vi "2.1.vi"() -> ()   [LabVIEW 2020]
uses:
  <vilib>/numeric/Random Number (Range) U64.vi
  <vilib>/numeric/sub_Random U32.vi
panel:
  out "Array 2":dbl[][](array[numeric])
  in  "Array":dbl[][](array[numeric])
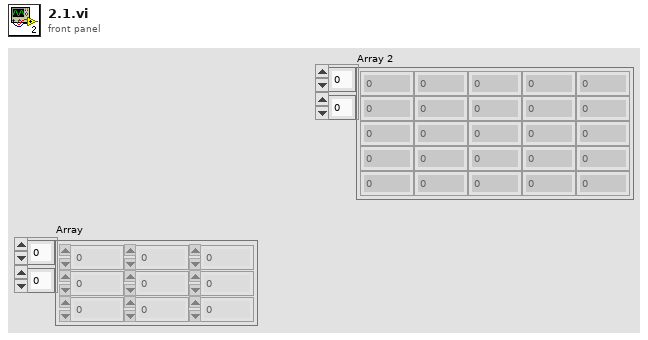
[diagram p1: front panel]
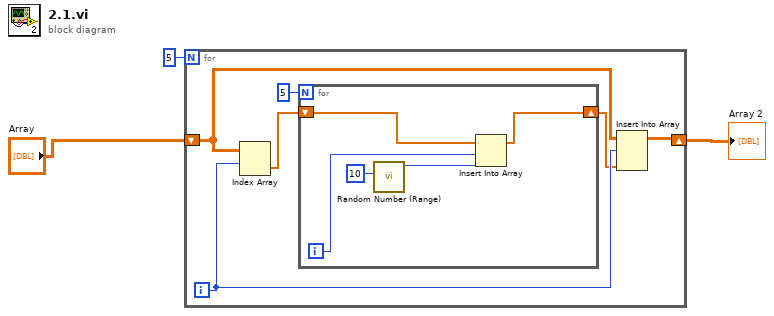
[diagram p0: block diagram]
diagram:
  n1 = for {
    N: 5 -> [_]
    shift-right: [w4] -> w1
    shift-left: "Array" -> [w6]
    i -> [w7]
    n2 = Index Array(array=w6, index (row)=w7) -> (element=w8:dbl[])  [unwired: 1 in]
    n3 = for {
      N: 5 -> [_]
      shift-right: [w10] -> w5
      shift-left: w8 -> [w13]
      i -> [w14]
      n4 = call-poly <vilib>:"Random Number (Range).vi"("lower bound (0)"=u64 10) -> ("number"=w11:u64)  [unwired: 10 in]
      n5 = Insert Into Array(array=w13, index=w14, new element=w11) -> (w10:dbl[])
    }
    n6 = Insert Into Array(array=w6, index (row)=w7, new element=w5) -> (w4:dbl[][])  [unwired: 1 in]
  }
  "Array 2" <- w1
